vi "TagDB Probe.vi"(11 "TagDB":refnum<k1>) -> (2 "Value String":string, 3 "Boolean":bool)   [LabVIEW 2017]
doc: "TagDB Library 2.0.1.6\nnevstop - NEVSTOP\nCopyright (c) 2018, NEVSTOP"
uses:
  TagDB/_Support/DataAccess/TagDB Ref to DVR.vi
  TagDB/_Support/Error/_[error50000]Invalid DB REF.vi
  TagDB/_Support/Error/_Build Error Cluster.vi
  TagDB/TagDB.lvlib
panel:
  out "Valid?":bool
  out "Name":string
  out "Last Item Change":timestamp format="%<%.3X>T"
  out "Last Data Change":timestamp format="%<%.3X>T"
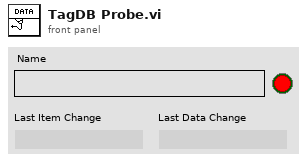
[diagram p1: front panel]
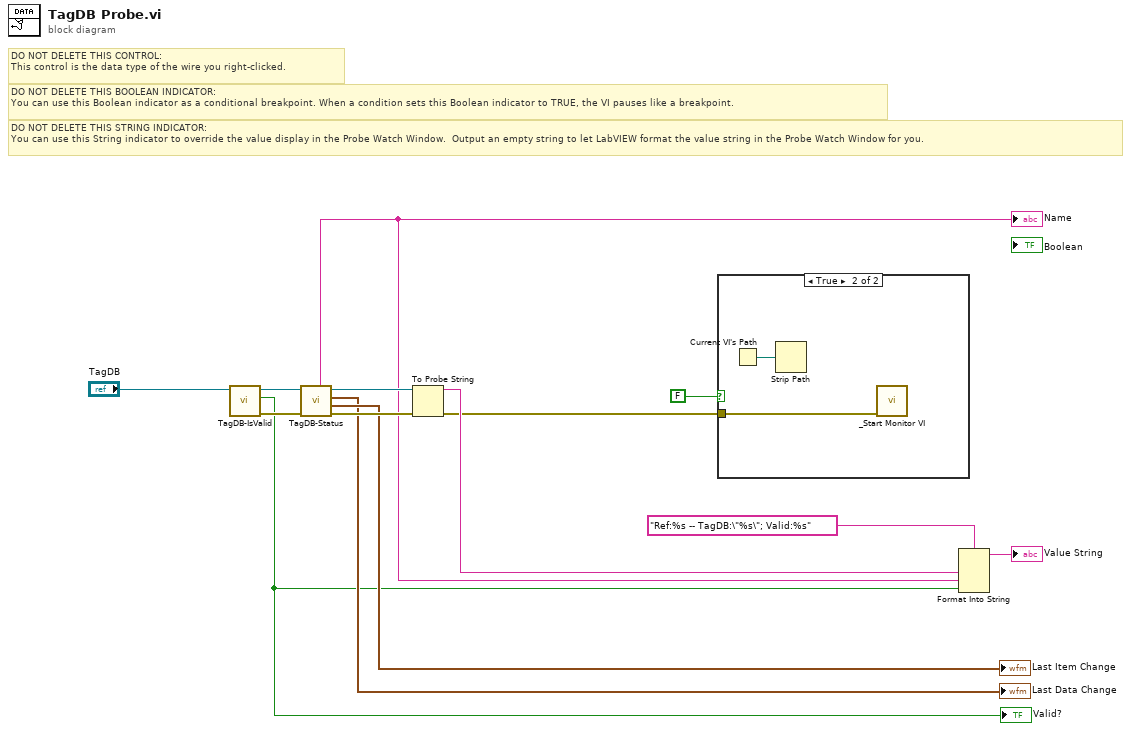
[diagram p0: block diagram]
diagram:
  # "DO NOT DELETE THIS STRING INDICATOR: \nYou can use this String indicator to override the value display in the Probe Watch Window.  Output an empty string to let LabVIEW format the value string in the Probe Watch Window for you."
  # "DO NOT DELETE THIS BOOLEAN INDICATOR: \nYou can use this Boolean indicator as a conditional breakpoint. When a condition sets this Boolean indicator to TRUE, the VI pauses like a breakpoint."
  # "DO NOT DELETE THIS CONTROL: \nThis control is the data type of the wire you right-clicked."
  n1 = call "TagDB-IsValid.vi"("TagDB"="TagDB") -> ("error out"=w12:errorcluster, "valid TagDB?"=w5:bool, "TagDB(dup)"=w13:refnum<k1>)  [unwired: 8 in]
  "Valid?" <- w5
  n2 = call "TagDB-Status.vi"("error in (no error)"=w12, "DB Ref"=w13) -> ("error out"=w11:errorcluster, "Item Change Timestamp"=→"Last Item Change":timestamp, "Global Change Timestamp"=→"Last Data Change":timestamp, "DB Ref(dup)"=w4:refnum<k1>, "db name"=w3:string)  [unwired: 4 in, 1 out]
  "Name" <- w3
  n3 = To Probe String(4:w11, 7:w4) -> (0:w2:errorcluster, 3:w8:string)  [unwired: 1 in]
  n4 = case shown="True" FALSE ("Start Monitoring Window") {
    tunnel: w2 -> [_ w16]
    frame False {
    }
    frame True {
      n5 = Current VI's Path() -> (path=w15:path)
      n6 = Strip Path(path=w15) -> ()  [unwired: 2 out]
      n7 = call "_Start Monitor VI.vi"("error in (no error)"=w16) -> ()  [unwired: 10 in, 1 out]
    }
  }
  n8 = Format Into String(format string="Ref:%s -- TagDB:\"%s\"; Valid:%s", w8, w3, w5) -> (resulting string=→"Value String":string)  [unwired: 2 in, 1 out]
